vi "Report.vi"() -> ()   [LabVIEW 2017]
uses:
  <vilib>/Utility/miscctls.llb/LVRowAndColumnUnsignedTypeDef.ctl
  a160b8e7-0040-4e34-a052-5f80b3aab475.vi
  <vilib>/addons/database/Connection.llb/DB Tools Open Connec (String).vi
  <vilib>/Utility/file.llb/Write Delimited Spreadsheet (string).vi
  Global/Global 1.vi
  <vilib>/regexp/Match Regular Expression.xnode
  <vilib>/addons/database/NI_Database_API.lvlib
  <vilib>/Utility/NIReport.llb/NI_report.lvclass
  <vilib>/Utility/NIReport.llb/Append Text Table to Report (wrap).vi
  <vilib>/Utility/miscctls.llb/LVRowAndColumnTypeDef.ctl
panel:
  out "reposr save header":string[](array[string])
  in  "SELECT REPORT TYPE":string(combo)="WITH TRECIABILITY"
  out "error out":errorcluster
  in  "error in (no error)":errorcluster
  in  "GET REPORT":bool
  in  "EXIT":bool
  in  "EXPORT TO EXCEL":bool
  in  "TO":timestamp format="%<%x>T"
  in  "FROM":timestamp format="%<%x>T"
  in  "BARCODE":string
  in  "TYPE":string(combo)="DATE TIME"
  in  "STATION WISE":string(combo)="0"
  out "Table":string[][](table)
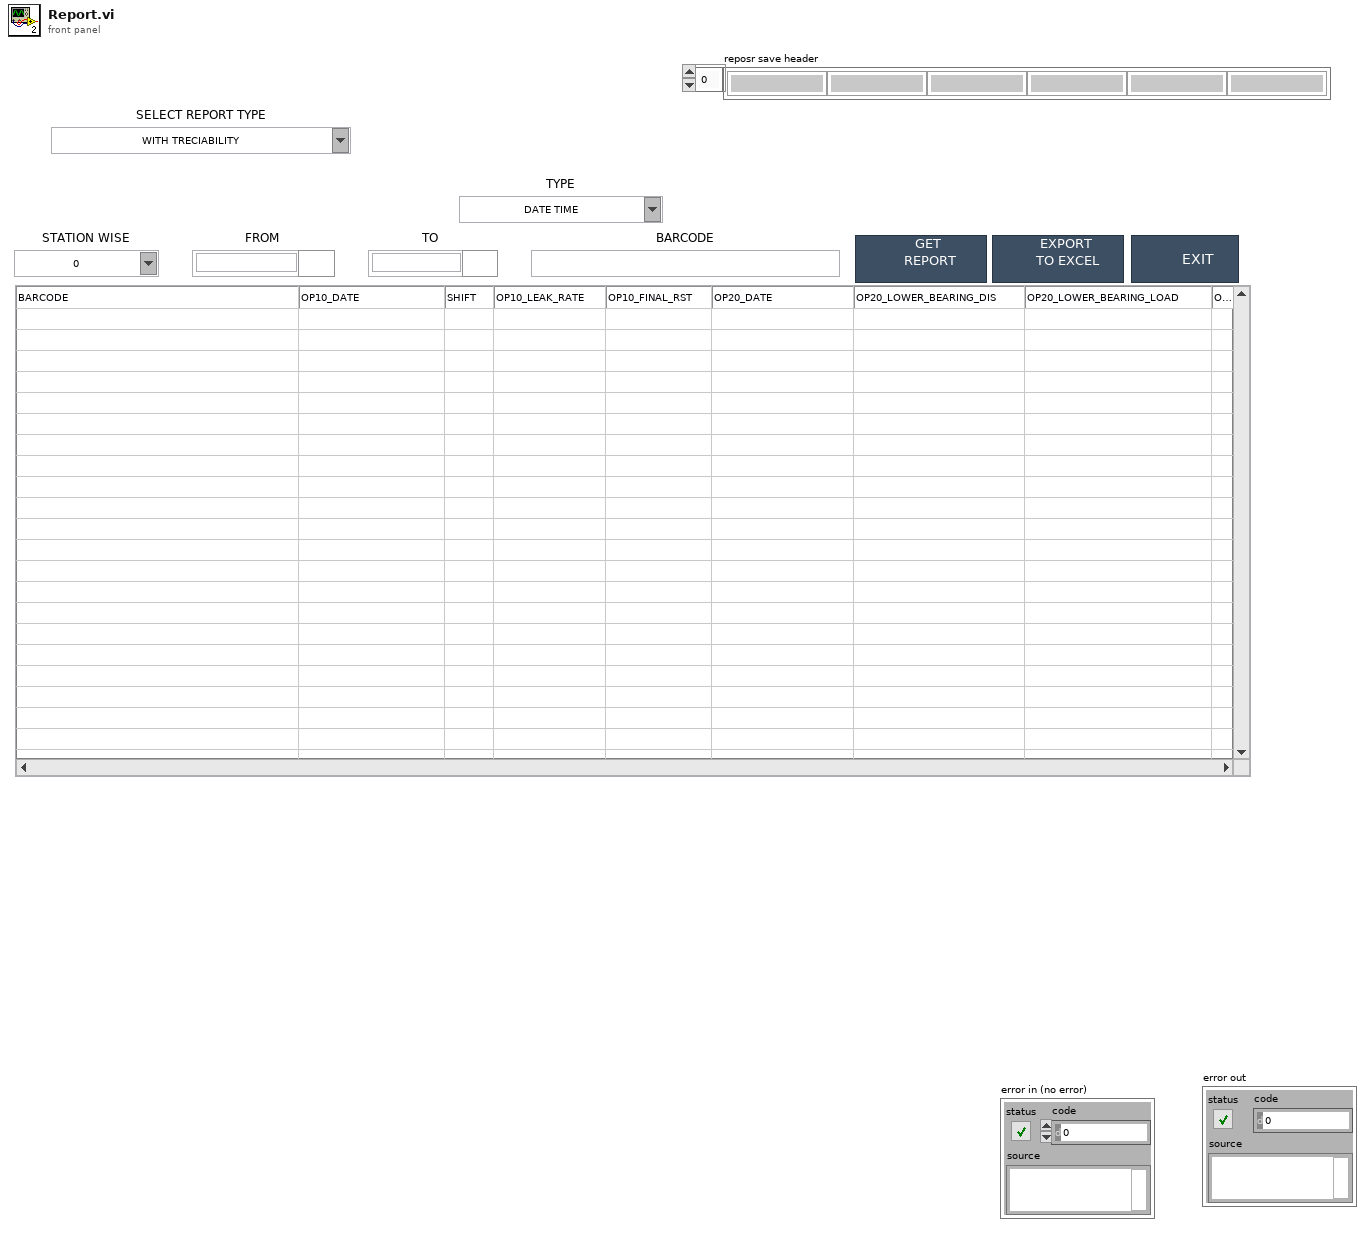
[diagram p1: front panel]
types:
  T1 = typedef "NI_Database_API.lvlib/Conn ObjectReference.ctl" = refnum<k1>
  T2 = typedef "LVRowAndColumnTypeDef.ctl" = cluster{"Row":i32, "Column":i32}
  T3 = typedef "LVRowAndColumnUnsignedTypeDef.ctl" = cluster{"Row":u32, "Column":u32}
  T4 = enum16{"Standard Report", "HTML", "Word", "Excel"}
  T5 = enum16{"maximized", "minimized", "normal", "no change"}
  T6 = enum32{"invalid app kind", "Development System", "Run Time System", "Student Edition", "Embedded LabVIEW", "Evaluation", "Custom"}
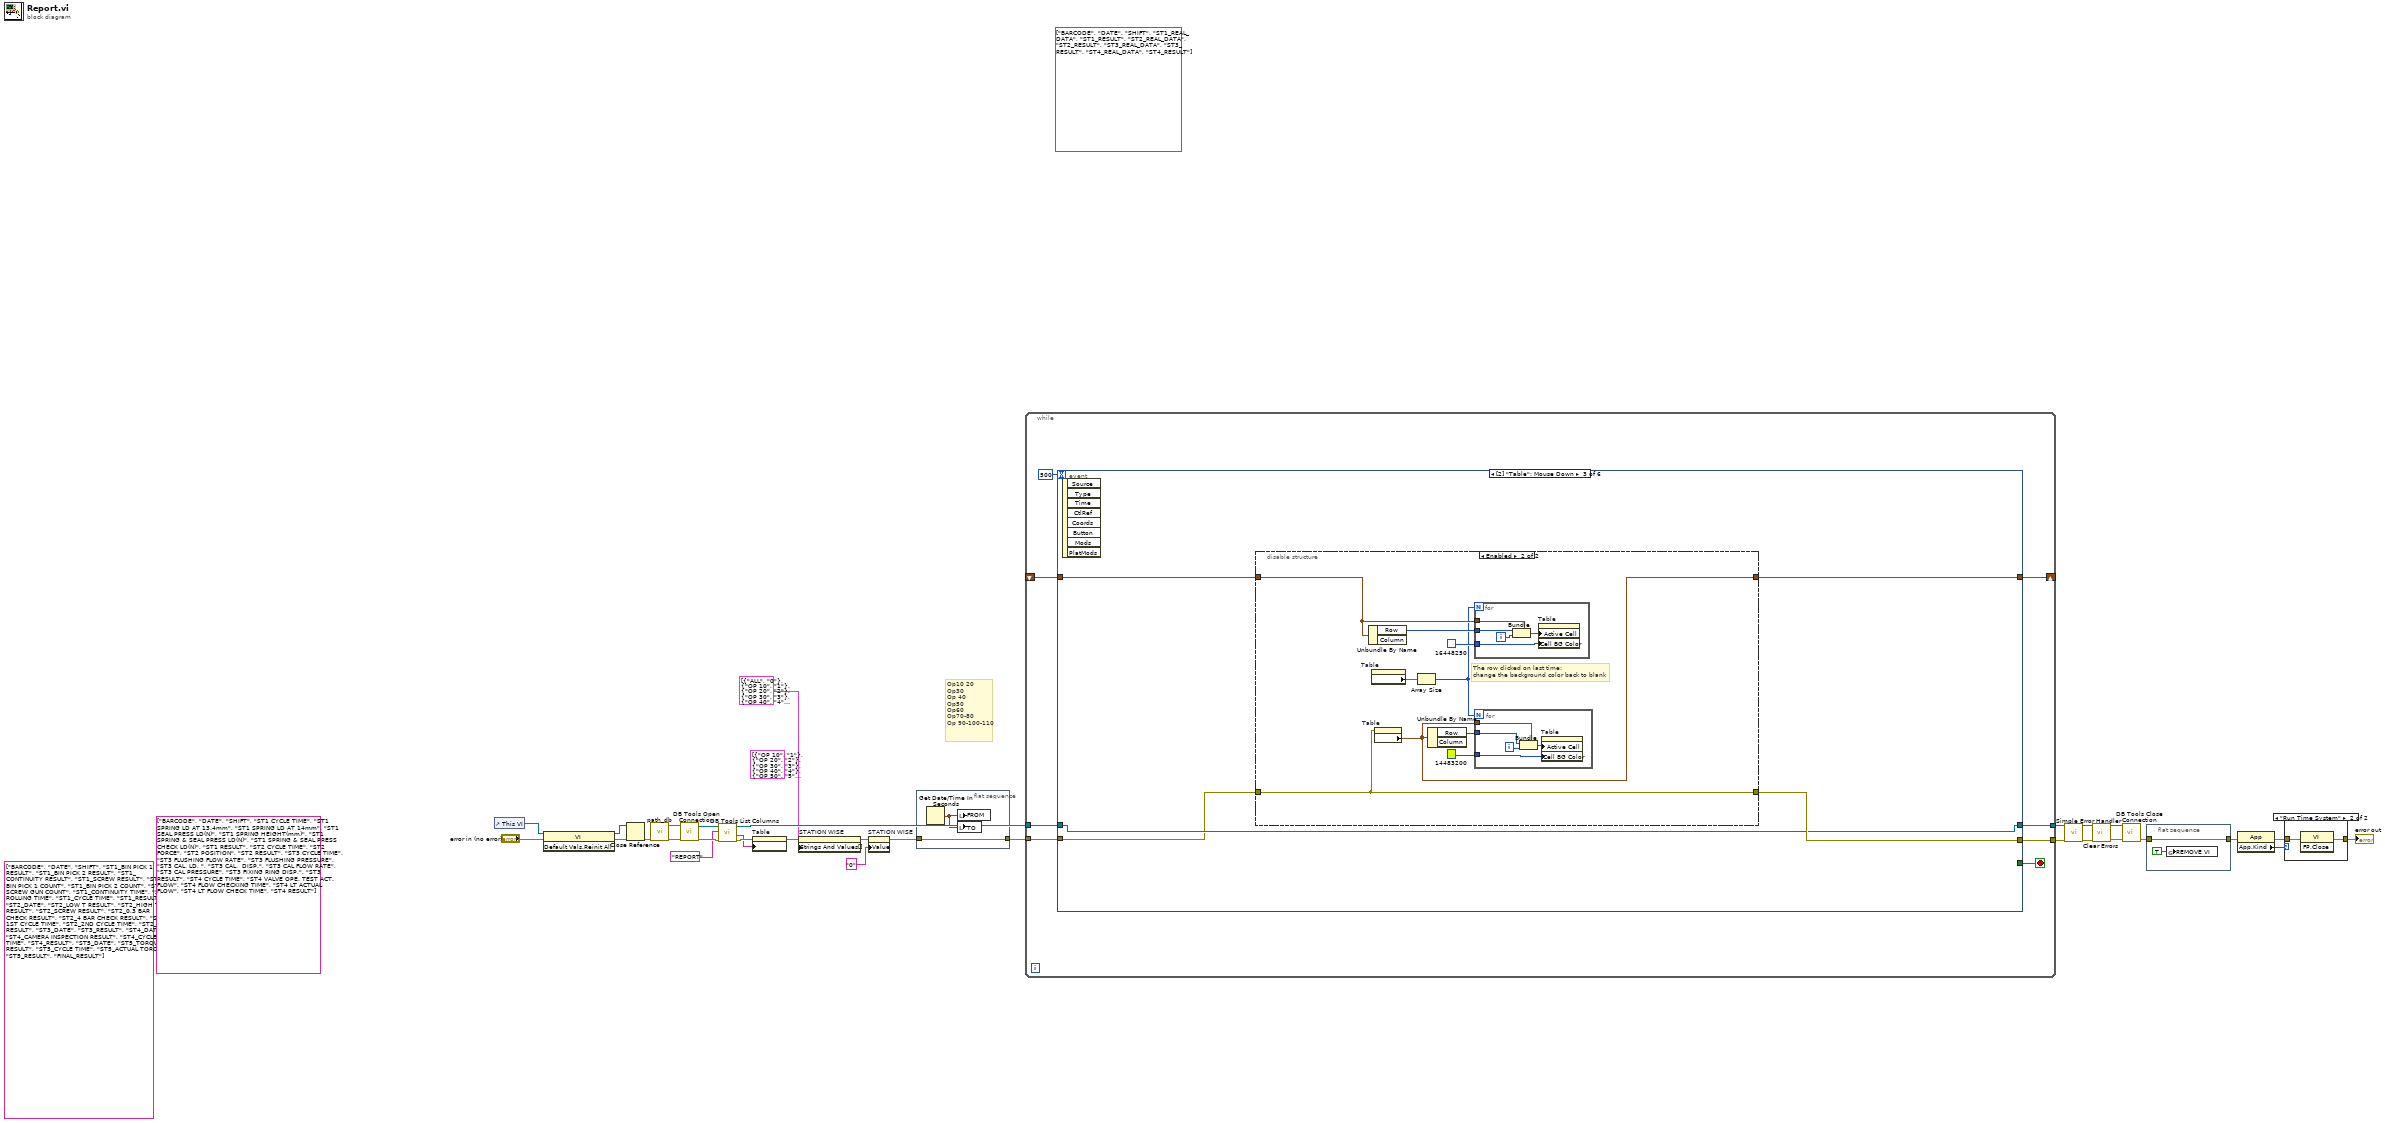
[diagram p0: block diagram]
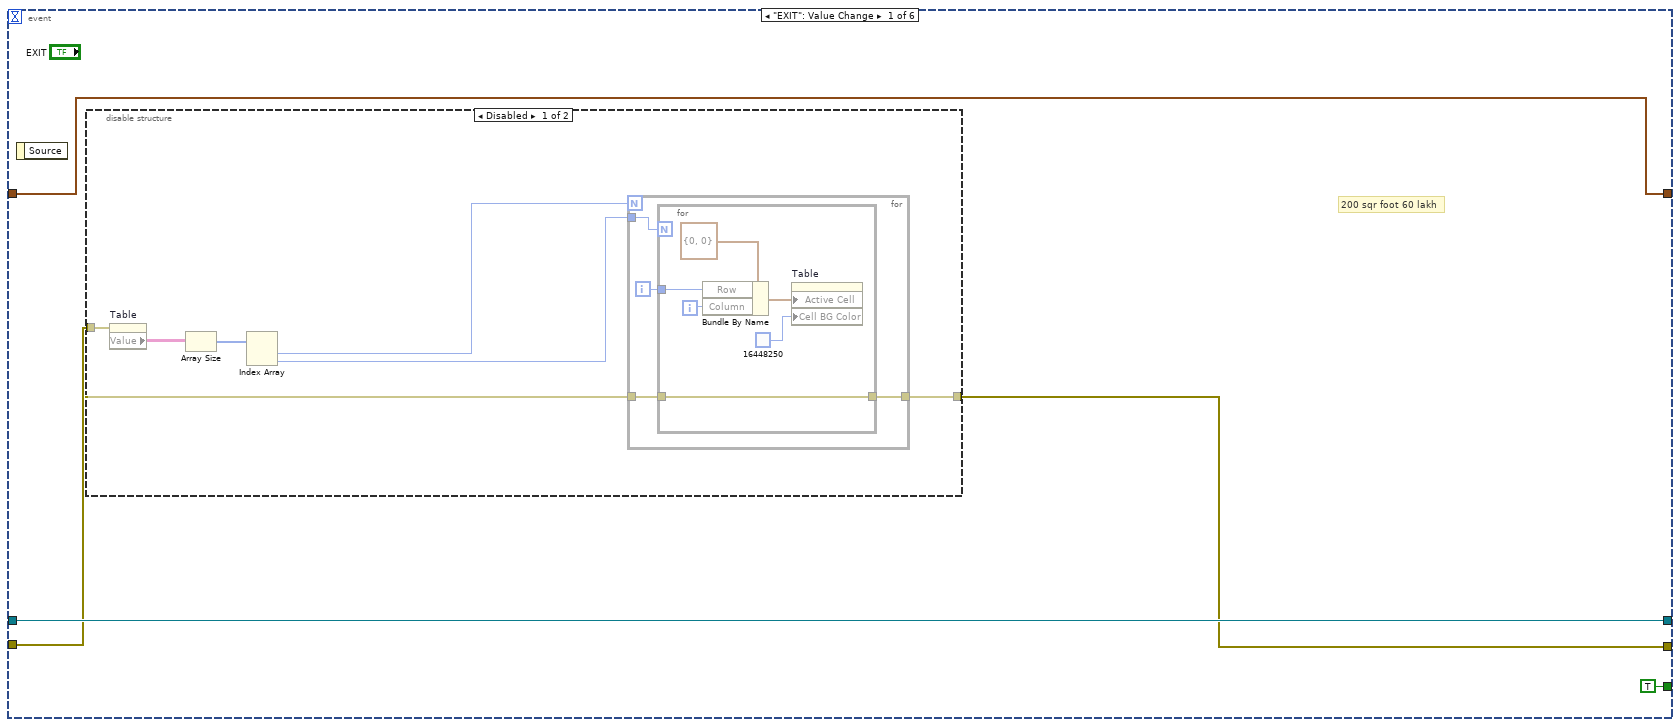
[diagram p2: hidden frame]
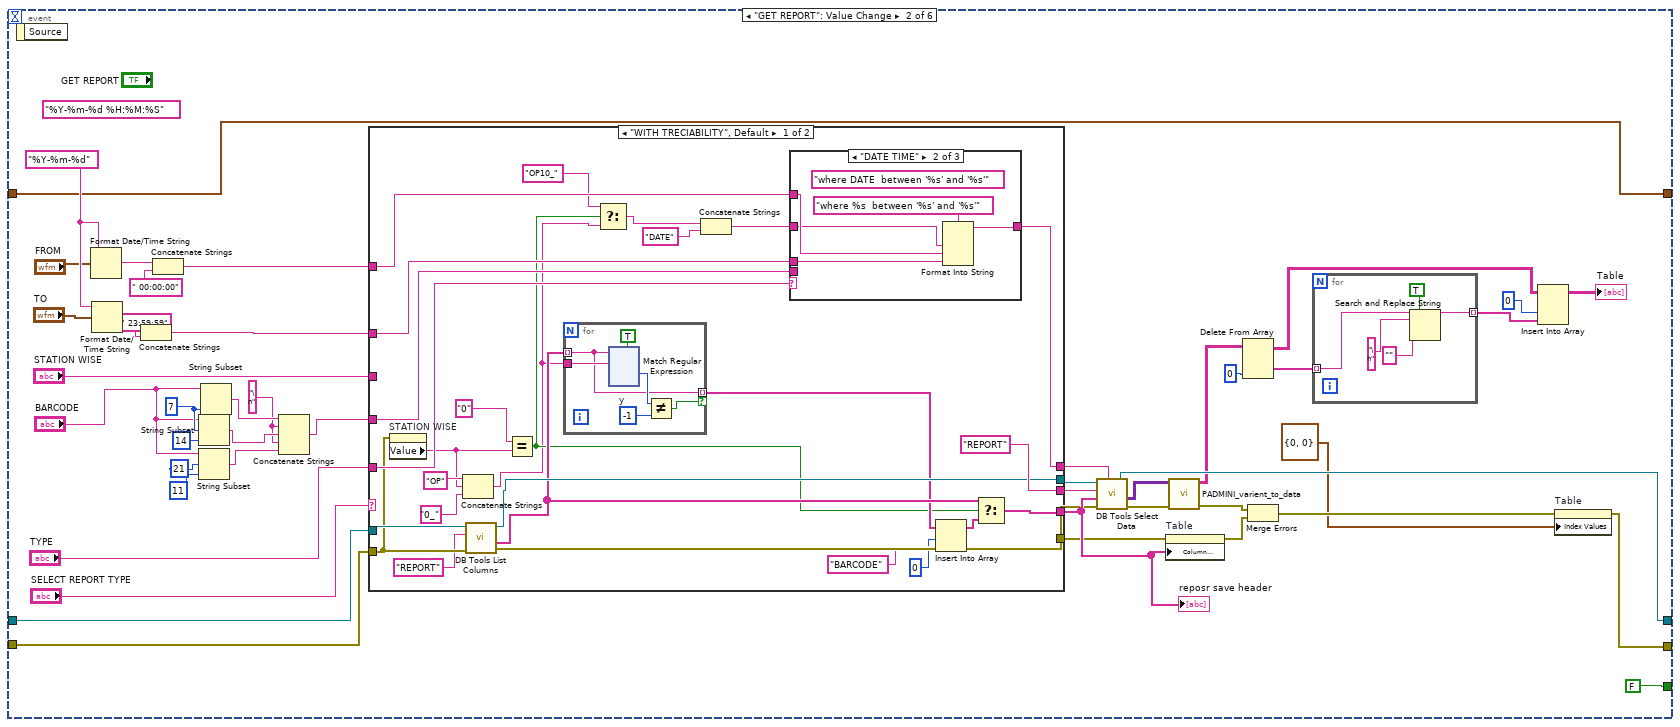
[diagram p4: hidden frame]
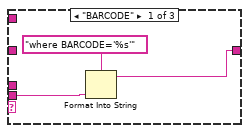
[diagram p5: hidden frame]
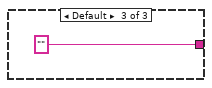
[diagram p6: hidden frame]
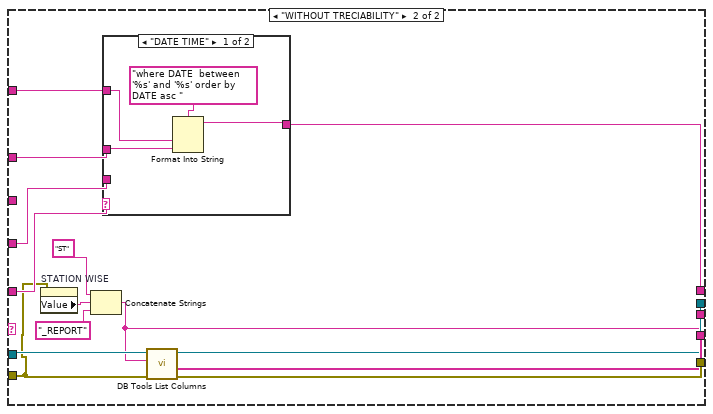
[diagram p7: hidden frame]
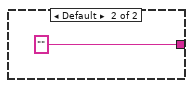
[diagram p8: hidden frame]
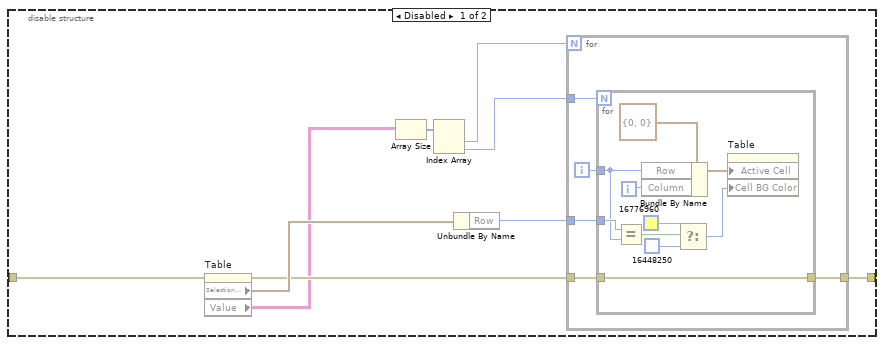
[diagram p9: hidden frame]
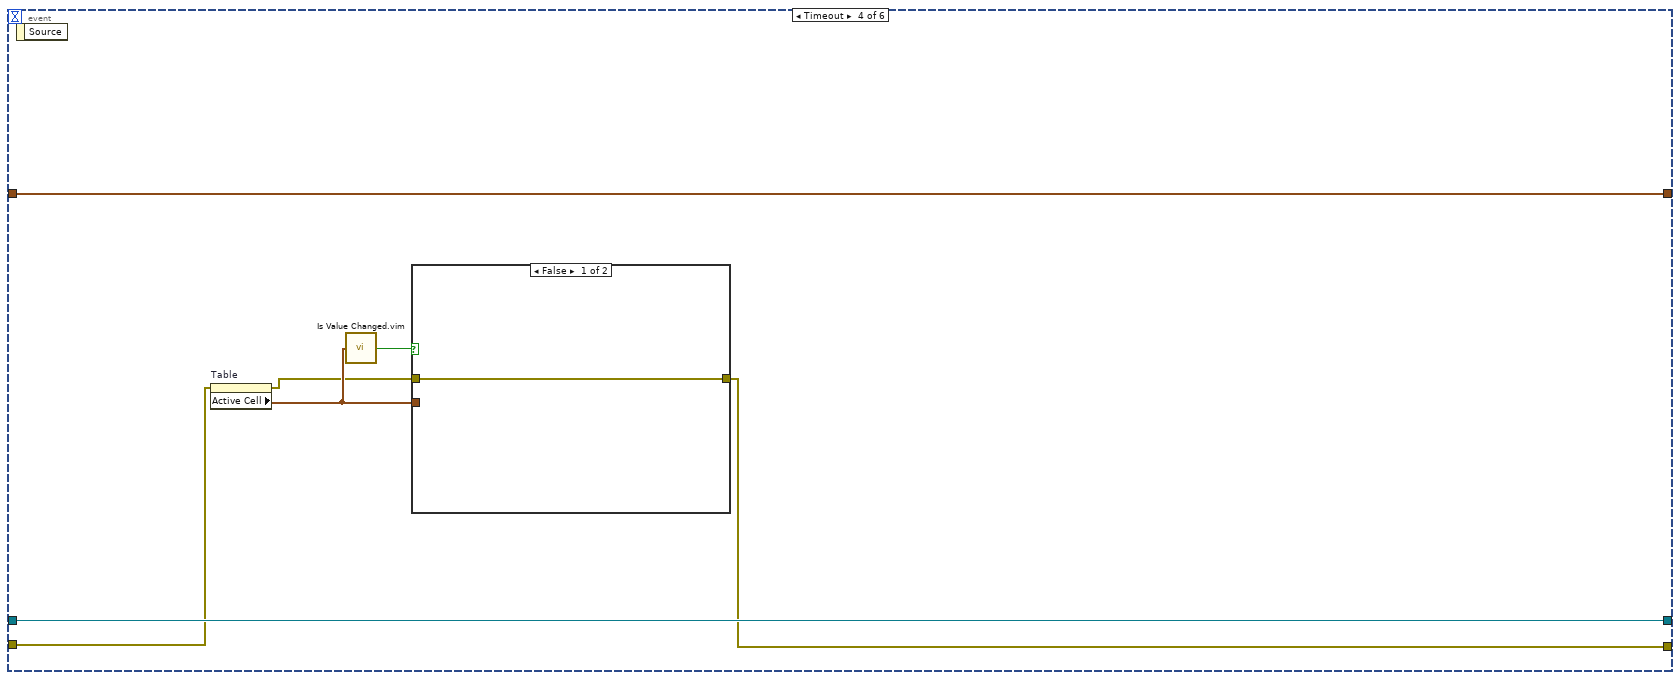
[diagram p10: hidden frame]
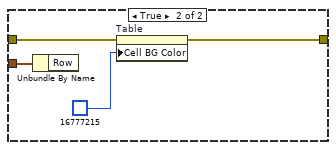
[diagram p11: hidden frame]
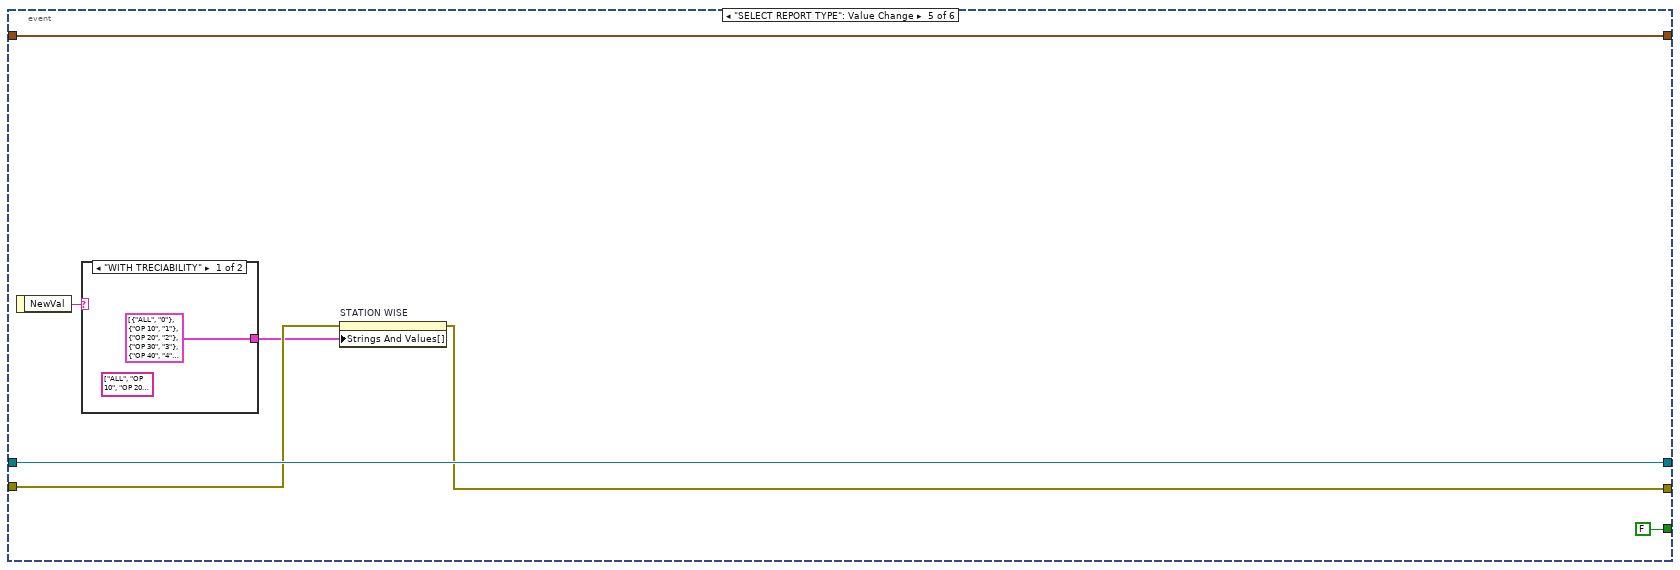
[diagram p12: hidden frame]
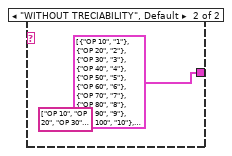
[diagram p13: hidden frame]
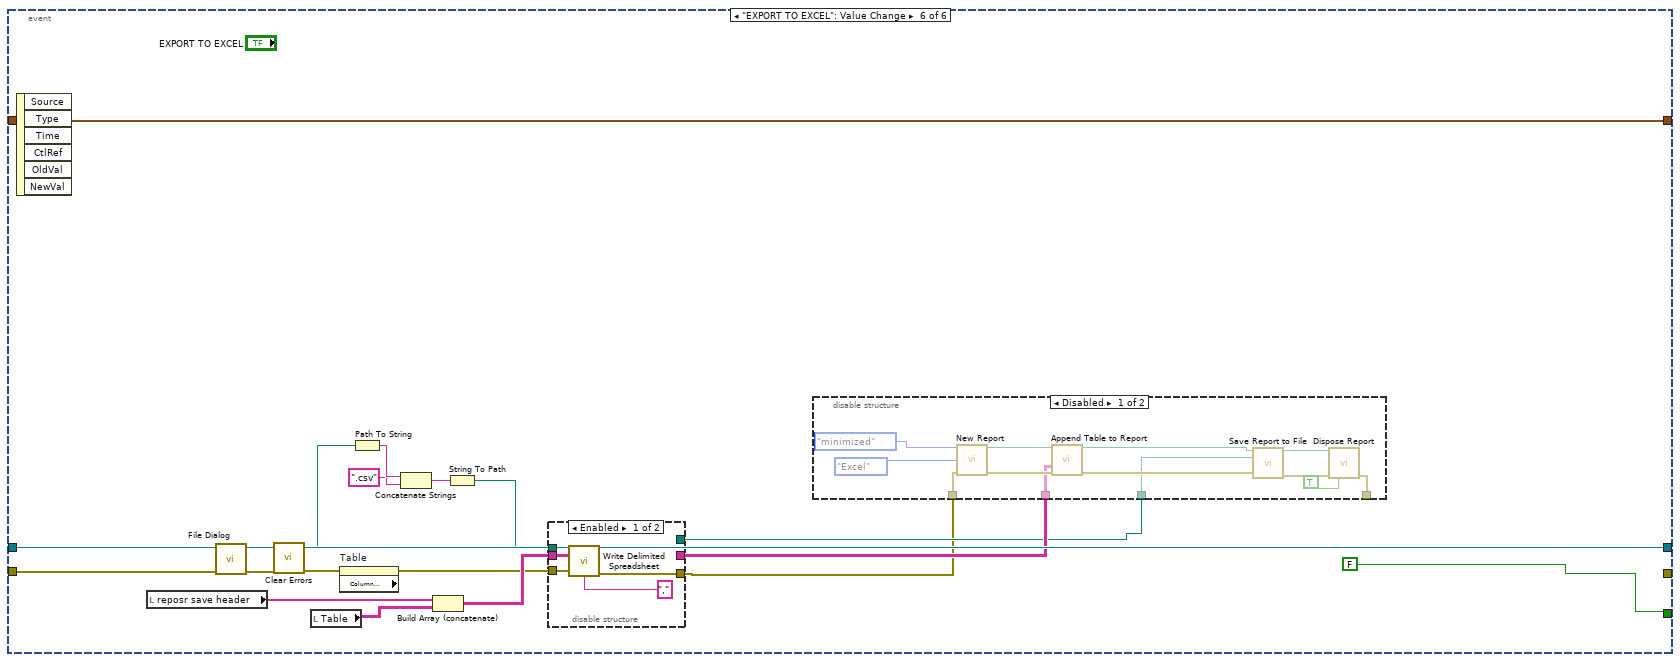
[diagram p14: hidden frame]
diagram:
  (unwired) cluster{"String":string, "Value":string}[] [{"String"="OP 10", "Value"="1"}, {"String"="OP 20", "Value"="2"}, {"String"="OP 30", "Value"="3"}, {"String"="OP 40", "Value"="4"}, {"String"="OP 50", "Value"="5"}, {"String"="OP 60", "Value"="6"}, {"String"="OP 70", "Value"="7"}, {"String"="OP 80", "Value"="8"}, {"String"="OP 90", "Value"="9"}, {"String"="OP 100", "Value"="10"}, {"String"="OP 110", "Value"="11"}] ("Strings And Values [] 2")
  (unwired) string[] ["BARCODE", "DATE", "SHIFT", "ST1_REAL_DATA", "ST1_RESULT", "ST2_REAL_DATA", "ST2_RESULT", "ST3_REAL_DATA", "ST3_RESULT", "ST4_REAL_DATA", "ST4_RESULT"]
  (unwired) string[] ["BARCODE", "DATE", "SHIFT", "ST1_BIN PICK 1 RESULT", "ST1_BIN PICK 2 RESULT", "ST1_CONTINUITY RESULT", "ST1_SCREW RESULT", "ST1_BIN PICK 1 COUNT", "ST1_BIN PICK 2 COUNT", "ST1_SCREW GUN COUNT", "ST1_CONTINUITY TIME", "ST1_ROLLING TIME", "ST1_CYCLE TIME", "ST1_RESULT", "ST2_DATE", "ST2_LOW T RESULT", "ST2_HIGH T RESULT", "ST2_SCREW RESULT", "ST2_0.3 BAR CHECK RESULT", "ST2_4 BAR CHECK RESULT", "ST2_1ST CYCLE TIME", "ST2_2ND CYCLE TIME", "ST2_RESULT", "ST3_DATE", "ST3_RESULT", "ST4_DATE", "ST4_CAMERA INSPECTION RESULT", "ST4_CYCLE TIME", "ST4_RESULT", "ST5_DATE", "ST5_TORQUE RESULT", "ST5_CYCLE TIME", "ST5_ACTUAL TORQUE", "ST5_RESULT", "FINAL_RESULT"]
  (unwired) string[] ["BARCODE", "DATE", "SHIFT", "ST1 CYCLE TIME", "ST1 SPRING LD AT 13.4mm", "ST1 SPRING LD AT 14mm", "ST1 SEAL PRESS LD(N)", "ST1 SPRING HEIGHT(mm)", "ST1 SPRING & SEAL PRESS LD(N)", "ST1 SPRING & SEAL PRESS CHECK LD(N)", "ST1 RESULT", "ST2 CYCLE TIME", "ST2 FORCE", "ST2 POSITION", "ST2 RESULT", "ST3 CYCLE TIME", "ST3 FLUSHING FLOW RATE", "ST3 FLUSHING PRESSURE", "ST3 CAL. LD. ", "ST3 CAL.  DISP.", "ST3 CAL FLOW RATE", "ST3 CAL PRESSURE", "ST3 FIXING RING DISP.", "ST3 RESULT", "ST4 CYCLE TIME", "ST4 VALVE OPE. TEST ACT. FLOW", "ST4 FLOW CHECKING TIME", "ST4 LT ACTUAL FLOW", "ST4 LT FLOW CHECK TIME", "ST4 RESULT"]
  # "Op10 20\nOp30\nOp 40\nOp50\nOp60\nOp70-80\nOp 90-100-110"
  n1 = control-ref of="This VI"() -> (w28:refnum<vi>)
  n2 = invoke class="VI" method="Default Vals.Reinit All"(reference=w28, error in="error in (no error)") -> (reference out=w26:refnum<vi>, error out=w25:errorcluster)  [unwired: 1 in, 1 out]
  n3 = Close Reference(reference=w26, error in (no error)=w25) -> (error out=w16:errorcluster)
  n4 = call "path_db.vi"("error in"=w16) -> ("error out"=w18:errorcluster, "resulting string"=w17:string)  [unwired: 9 in]
  n5 = call-poly <vilib>:"DB Tools Open Connection.vi"("error in (no error)"=w18, "connection information"=w17) -> ("error out"=w11:errorcluster, "connection reference"=w8:T1)  [unwired: 6 in]
  n6 = call <vilib>:"DB Tools List Columns.vi"("error in (no error)"=w11, "table"="REPORT", "connection reference"=w8) -> ("error out"=w10:errorcluster, "columns"=w7:string[], "connection reference out"=w9:T1)  [unwired: 1 in, 1 out]
  n7 = property on="Table" class="Tbl (strict)"(error in=w10, "Column Headers[]"=w7) -> (error out=w13:errorcluster)  [unwired: 1 in, 1 out]
  n8 = property on="STATION WISE" class="CmbBox"(error in=w13, "Strings And Values[]"=cluster{"String":string, "Value":string}[] [{"String"="ALL", "Value"="0"}, {"String"="OP 10", "Value"="1"}, {"String"="OP 20", "Value"="2"}, {"String"="OP 30", "Value"="3"}, {"String"="OP 40", "Value"="4"}, {"String"="OP 50", "Value"="5"}, {"String"="OP 60", "Value"="6"}, {"String"="OP 70", "Value"="7"}, {"String"="OP 80", "Value"="8"}, {"String"="OP 90", "Value"="9"}, {"String"="OP 100", "Value"="10"}, {"String"="OP 110", "Value"="11"}] ("Strings And Values [] 2")) -> (error out=w5:errorcluster)  [unwired: 1 in, 1 out]
  n9 = property on="STATION WISE" class="CmbBox"(error in=w5, "Value"="0") -> (error out=w4:errorcluster)  [unwired: 1 in, 1 out]
  n10 = flat-sequence {
    tunnel: w4 -> [w29]
    tunnel: [w29] -> w12
    frame #0 {
      n11 = Get Date/Time In Seconds() -> (seconds since 1Jan1904=w30:timestamp)
      n12 = local write "FROM"(w30) -> ()
      n13 = local write "TO"(w30) -> ()
    }
  }
  n14 = while {
    tunnel: [w35] -> w1
    tunnel: w12 -> [w37]
    tunnel: w9 -> [w36]
    tunnel: [w34] -> w14
    shift-right: [w32] -> _
    shift-left: _ -> [w31]
    stop <- w38 stop-if-true
    n15 = event shown="[2] \"Table\": Mouse Down" {
      selector: _ -> [_ _ _ _ _ _]
      dyn-events: _ -> [_ _ _ _ _ _]
      timeout: 500 -> [_ _ _ _ _ _]
      tunnel: [TRUE FALSE _ _ FALSE FALSE] -> w38
      tunnel: w37 -> [w41 w84 w288 w337 w350 w360]
      tunnel: w36 -> [w42 w82 w289 w340 w352 w371]
      tunnel: [w42 w90 w289 w340 w352 w371] -> w34
      tunnel: [w40 w71 w290 w335 w347 _] -> w35
      tunnel: [w39 w70 w287 w334 w346 w355] -> w32
      tunnel: w31 -> [w39 w70 w286 w334 w346 w355]
      event "EXIT": Value Change {
        # "200 sqr foot 60 lakh"
        n16 = event-data() -> ()  [unwired: 1 in, 1 out]
        n17 = disable-structure shown="Disabled" {
          disable-tunnel: w41 -> [w49 _]
          disable-tunnel: [w48 _] -> w40
          frame Disabled {
            n18 = property on="Table" class="Tbl (strict)"(error in=w49) -> ("Value"=w47:string[][])  [unwired: 1 in, 2 out]
            n19 = Array Size(array=w47) -> (size(s)=w46:i32[])
            n20 = Index Array(array=w46) -> (element #1=w45:i32, element #2=w44:i32)  [unwired: 2 in]
            n21 = for {
              N: w45 -> [_]
              tunnel: w44 -> [w53]
              tunnel: [w50] -> w48
              tunnel: w49 -> [w51]
              i -> [w52]
              n22 = for {
                N: w53 -> [_]
                tunnel: w52 -> [w56]
                tunnel: w51 -> [w55]
                tunnel: [w55] -> w50
                i -> [w57]
                n23 = Bundle By Name(cluster=T2 {"Row"=0, "Column"=0} ("Selection Start 2"), "Row"=w56, "Column"=w57) -> (w58:T2)
                n24 = property on="Table" class="Tbl (strict)"("Active Cell"=w58, "Cell BG Color"=u32 16448250) -> ()  [unwired: 2 in, 2 out]
              }
            }
          }
          frame Enabled {
          }
        }
      }
      event "GET REPORT": Value Change {
        w62 = "\n"
        w69 = 7 ("line index")
        (unwired) "%Y-%m-%d %H:%M:%S" ("time format string (%c)")
        w103 = "%Y-%m-%d" ("time format string (%c)")
        n25 = event-data() -> ()  [unwired: 1 in, 1 out]
        n26 = Format Date/Time String(time format string (%c)=w103, seconds (now)="FROM") -> (date/time string=w97:string)  [unwired: 1 in]
        n27 = Format Date/Time String(time format string (%c)=w103, seconds (now)="TO") -> (date/time string=w94:string)  [unwired: 1 in]
        n28 = Concatenate Strings(w94, " 23:59:59" ("time format string (%c)")) -> (w93:string)
        n29 = Concatenate Strings(w97, " 00:00:00" ("time format string (%c)")) -> (w96:string)
        n30 = String Subset(string="BARCODE", offset (0)=w69, length (rest)=14 ("line index")) -> (substring=w64:string)
        n31 = String Subset(string="BARCODE", offset (0)=21 ("line index"), length (rest)=11 ("line index")) -> (substring=w63:string)
        n32 = String Subset(string="BARCODE", length (rest)=w69) -> (substring=w65:string)  [unwired: 1 in]
        n33 = Concatenate Strings(w65, w62, w64, w62, w63) -> (w61:string)
        n34 = case shown="\"WITH TRECIABILITY\", Default" "SELECT REPORT TYPE" {
          tunnel: "TYPE" -> [w137 w280]
          tunnel: [w136 w279] -> w104
          tunnel: w61 -> [w135 w278]
          tunnel: w96 -> [w134 w277]
          tunnel: w93 -> [w119 w273]
          tunnel: "STATION WISE" -> [_ _]
          tunnel: ["REPORT" w268] -> w85
          tunnel: w84 -> [w125 w267]
          tunnel: [w130 w272] -> w79
          tunnel: [w117 w271] -> w83
          tunnel: w82 -> [w132 w270]
          tunnel: [w131 w269] -> w81
          frame "WITH TRECIABILITY", Default {
            n35 = property on="STATION WISE" class="CmbBox"(error in=w125) -> ("Value"=w120:string)  [unwired: 1 in, 2 out]
            n36 = Concatenate Strings("OP" ("element"), w120, "0_" ("element")) -> (w112:string)
            n37 = call <vilib>:"DB Tools List Columns.vi"("error in (no error)"=w125, "table"="REPORT", "connection reference"=w132) -> ("error out"=w130:errorcluster, "columns"=w124:string[], "connection reference out"=w131:T1)  [unwired: 1 in, 1 out]
            n38 = Equal?(x="0", y=w120) -> (x = y?=w114:bool)
            n39 = for {
              tunnel: w124 -> [w139] mode=indexing
              tunnel: w112 -> [w143]
              tunnel: [w139] -> w118 mode=indexing if=w138
              w140 = -1  # y
              n40 = xnode "Match Regular Expression"("input string"=w139, "regular expression"=w143, "multiline? (F)"=TRUE) -> ("offset past match"=w141:i32)  [unwired: 3 in, 4 out]
              n41 = Not Equal?(x=w141, y=w140) -> (x != y?=w138:bool)
            }
            n42 = Select(t="OP10_", s=w114, f=w112) -> (s? t:f=w111:string)
            n43 = Concatenate Strings(w111, "DATE") -> (w115:string)
            n44 = case shown="\"DATE TIME\"" w137 {
              tunnel: [w259 w264 ""] -> w136
              tunnel: w135 -> [w258 _ _]
              tunnel: w134 -> [_ w263 _]
              tunnel: w119 -> [_ w262 _]
              tunnel: w115 -> [_ w261 _]
              frame "BARCODE" {
                n45 = Format Into String(format string="where BARCODE='%s'", w258) -> (resulting string=w259:string)  [unwired: 2 in, 1 out]
              }
              frame "DATE TIME" {
                (unwired) "where DATE  between '%s' and '%s'"
                n46 = Format Into String(format string="where %s  between '%s' and '%s'", w261, w263, w262) -> (resulting string=w264:string)  [unwired: 2 in, 1 out]
              }
              frame Default {
              }
            }
            n47 = Insert Into Array(array=w118, index=0, new element="BARCODE" ("String")) -> (w128:string[])
            n48 = Select(t=w124, s=w114, f=w128) -> (s? t:f=w117:string[])
          }
          frame "WITHOUT TRECIABILITY" {
            n49 = property on="STATION WISE" class="CmbBox"(error in=w267) -> ("Value"=w276:string)  [unwired: 1 in, 2 out]
            n50 = Concatenate Strings("ST", w276, "_REPORT") -> (w268:string)
            n51 = case shown="\"DATE TIME\"" w280 {
              tunnel: [w284 ""] -> w279
              tunnel: w278 -> [_ _]
              tunnel: w277 -> [w283 _]
              tunnel: w273 -> [w282 _]
              frame "DATE TIME" {
                n52 = Format Into String(format string="where DATE  between '%s' and '%s' order by DATE asc ", w283, w282) -> (resulting string=w284:string)  [unwired: 2 in, 1 out]
              }
              frame Default {
              }
            }
            n53 = call <vilib>:"DB Tools List Columns.vi"("error in (no error)"=w267, "table"=w268, "connection reference"=w270) -> ("error out"=w272:errorcluster, "columns"=w271:string[], "connection reference out"=w269:T1)  [unwired: 1 in, 1 out]
          }
        }
        "reposr save header" <- w83
        n54 = call <vilib>:"DB Tools Select Data.vi"("condition"=w104, "error in (no error)"=w79, "columns"=w83, "table"=w85, "connection reference"=w81) -> ("error out"=w88:errorcluster, "data"=w92:variant[][], "connection reference out"=w90:T1)  [unwired: 1 in]
        n55 = property on="Table" class="Tbl (strict)"(error in=w79, "Column Headers[]"=w83) -> (error out=w87:errorcluster)  [unwired: 1 in, 1 out]
        n56 = call "PADMINI_varient_to_data.vi"("error in (no error)"=w88, "data"=w92) -> ("error out"=w86:errorcluster, "Array"=w74:string[][])  [unwired: 8 in]
        n57 = Delete From Array(array=w74, index (col)=0 ("disabled index (col)")) -> (deleted portion=w77:string[], array with subset deleted=w75:string[][])  [unwired: 2 in]
        n58 = Merge Errors(w86, w87) -> (w91:errorcluster)
        n59 = for {
          tunnel: w77 -> [w107] mode=indexing
          tunnel: [w106] -> w76 mode=indexing
          n60 = Search and Replace String(replace all?=TRUE ("replace all? (F)"), input string=w107, search string="\n", replace string="" ("replace string (\"\")")) -> (result string=w106:string)  [unwired: 4 in, 3 out]
        }
        n61 = Insert Into Array(array=w75, index (col)=0 ("disabled index (col)"), new element=w76) -> (→"Table":string[][])  [unwired: 1 in]
        n62 = property on="Table" class="Tbl (strict)"(error in=w91, "Index Values"=T3 {"Row"=0, "Column"=0}) -> (error out=w71:errorcluster)  [unwired: 1 in, 1 out]
      }
      event "Table": Mouse Down {
        n63 = event-data() -> ()  [unwired: 1 in, 8 out]
        n64 = disable-structure shown="Enabled" {
          disable-tunnel: [w299 w317] -> w290
          disable-tunnel: w288 -> [w296 w317]
          disable-tunnel: [_ w318] -> w287
          disable-tunnel: w286 -> [_ w319]
          frame Disabled {
            n65 = property on="Table" class="Tbl (strict)"(error in=w296) -> (error out=w295:errorcluster, "Selection Start"=w297:T2, "Value"=w293:string[][])  [unwired: 1 in, 1 out]
            n66 = Array Size(array=w293) -> (size(s)=w294:i32[])
            n67 = Index Array(array=w294) -> (element #1=w291:i32, element #2=w292:i32)  [unwired: 2 in]
            n68 = Unbundle By Name(w297) -> ("Row"=w298:i32)
            n69 = for {
              N: w291 -> [_]
              tunnel: w298 -> [w302]
              tunnel: w292 -> [w304]
              tunnel: [w300] -> w299
              tunnel: w295 -> [w301]
              i -> [w303]
              n70 = for {
                N: w304 -> [_]
                tunnel: w303 -> [w310]
                tunnel: w302 -> [w311]
                tunnel: w301 -> [w305]
                tunnel: [w305] -> w300
                i -> [w312]
                n71 = Equal?(x=w311, y=w310) -> (x = y?=w309:bool)
                n72 = Bundle By Name(cluster=T2 {"Row"=0, "Column"=0} ("Selection Start 2"), "Row"=w310, "Column"=w312) -> (w313:T2)
                n73 = Select(t=u32 16776960, s=w309, f=u32 16448250) -> (s? t:f=w306:u32)
                n74 = property on="Table" class="Tbl (strict)"("Active Cell"=w313, "Cell BG Color"=w306) -> ()  [unwired: 2 in, 2 out]
              }
            }
          }
          frame Enabled {
            # "The row clicked on last time:\nchange the background color back to blank"
            n75 = Unbundle By Name(w319) -> ("Row"=w321:i32)  [unwired: 1 out]
            n76 = property on="Table" class="Tbl (strict)"() -> ("Column Headers[]"=w316:string[])  [unwired: 2 in, 2 out]
            n77 = property on="Table" class="Tbl (strict)"(error in=w317) -> ("Selection Start"=w318:T2)  [unwired: 1 in, 2 out]
            n78 = Array Size(array=w316) -> (size(s)=w315:i32)
            n79 = Unbundle By Name(w318) -> ("Row"=w322:i32)  [unwired: 1 out]
            n80 = for {
              N: w315 -> [_]
              tunnel: u32 16448250 -> [w328]
              tunnel: w319 -> [w327]
              tunnel: w321 -> [w326]
              i -> [w325]
              n81 = Bundle(cluster=w327, "Row"=w326, "Column"=w325) -> (w324:T2)
              n82 = property on="Table" class="Tbl (strict)"("Active Cell"=w324, "Cell BG Color"=w328) -> ()  [unwired: 2 in, 2 out]
            }
            n83 = for {
              N: w315 -> [_]
              tunnel: u32 14483200 -> [w333]
              tunnel: w318 -> [w332]
              tunnel: w322 -> [w331]
              i -> [w330]
              n84 = Bundle(cluster=w332, "Row"=w331, "Column"=w330) -> (w329:T2)
              n85 = property on="Table" class="Tbl (strict)"("Active Cell"=w329, "Cell BG Color"=w333) -> ()  [unwired: 2 in, 2 out]
            }
          }
        }
      }
      event Timeout {
        n86 = event-data() -> ()  [unwired: 1 in, 1 out]
        n87 = property on="Table" class="Tbl (strict)"(error in=w337) -> (error out=w336:errorcluster, "Active Cell"=w339:T2)  [unwired: 1 in, 1 out]
        n88 = call "Is Value Changed.vim"("value"=w339) -> ("changed or first call?"=w338:bool)
        n89 = case shown="False" w338 {
          tunnel: w339 -> [_ w345]
          tunnel: w336 -> [w341 w343]
          tunnel: [w341 w342] -> w335
          frame False {
          }
          frame True {
            n90 = Unbundle By Name(w345) -> ()  [unwired: 1 out]
            n91 = property on="Table" class="Tbl (strict)"(error in=w343, "Cell BG Color"=u32 16777215) -> (error out=w342:errorcluster)  [unwired: 1 in, 1 out]
          }
        }
      }
      event "SELECT REPORT TYPE": Value Change {
        n92 = event-data() -> ("NewVal"=w351:string)  [unwired: 1 in]
        n93 = case shown="\"WITH TRECIABILITY\"" w351 {
          tunnel: [cluster{"String":string, "Value":string}[] [{"String"="ALL", "Value"="0"}, {"String"="OP 10", "Value"="1"}, {"String"="OP 20", "Value"="2"}, {"String"="OP 30", "Value"="3"}, {"String"="OP 40", "Value"="4"}, {"String"="OP 50", "Value"="5"}, {"String"="OP 60", "Value"="6"}, {"String"="OP 70", "Value"="7"}, {"String"="OP 80", "Value"="8"}, {"String"="OP 90", "Value"="9"}, {"String"="OP 100", "Value"="10"}, {"String"="OP 110", "Value"="11"}] ("Strings And Values [] 2") cluster{"String":string, "Value":string}[] [{"String"="OP 10", "Value"="1"}, {"String"="OP 20", "Value"="2"}, {"String"="OP 30", "Value"="3"}, {"String"="OP 40", "Value"="4"}, {"String"="OP 50", "Value"="5"}, {"String"="OP 60", "Value"="6"}, {"String"="OP 70", "Value"="7"}, {"String"="OP 80", "Value"="8"}, {"String"="OP 90", "Value"="9"}, {"String"="OP 100", "Value"="10"}, {"String"="OP 110", "Value"="11"}] ("Strings And Values [] 2")] -> w348
          frame "WITH TRECIABILITY" {
            (unwired) string[] ["ALL", "OP 10", "OP 20", "OP 30", "OP 40", "OP 50", "OP 60", "OP 70", "OP 80", "OP 90", "OP 100", "OP 110"] ("Strings []")
          }
          frame "WITHOUT TRECIABILITY", Default {
            (unwired) string[] ["OP 10", "OP 20", "OP 30", "OP 40", "OP 50", "OP 60", "OP 70", "OP 80", "OP 90", "OP 100", "OP 110"] ("Strings []")
          }
        }
        n94 = property on="STATION WISE" class="CmbBox"(error in=w350, "Strings And Values[]"=w348) -> (error out=w347:errorcluster)  [unwired: 1 in, 1 out]
      }
      event "EXPORT TO EXCEL": Value Change {
        n95 = event-data() -> ()  [unwired: 1 in, 6 out]
        n96 = local read "reposr save header"() -> (w356:string[])
        n97 = call "File Dialog"("error in"=w360) -> ("selected path"=w369:path, "error out"=w370:errorcluster)  [unwired: 11 in, 2 out]
        n98 = call <vilib>:"Clear Errors.vi"("error in (no error)"=w370) -> ("error out"=w363:errorcluster)  [unwired: 5 in, 1 out]
        n99 = local read "Table"() -> (w372:string[][])
        n100 = property on="Table" class="Tbl (strict)" props=["Column Headers[]"](error in=w363) -> (error out=w362:errorcluster)  [unwired: 1 in, 2 out]
        n101 = Path To String(path=w369) -> (string=w368:string)
        n102 = Concatenate Strings(w368, ".csv" ("string")) -> (w366:string)
        n103 = Build Array (concatenate)(w356, w372) -> (w364:string[][])
        n104 = String To Path(string=w366) -> (path=w365:path)
        n105 = disable-structure shown="Enabled" {
          disable-tunnel: w365 -> [w391 w392]
          disable-tunnel: [w390 w394] -> w357
          disable-tunnel: w364 -> [w389 w393]
          disable-tunnel: w362 -> [w387 w394]
          disable-tunnel: [_ w393] -> w359
          disable-tunnel: [_ w392] -> w358
          frame Enabled {
            n106 = call-poly <vilib>:"Write Delimited Spreadsheet.vi"("file path (dialog if empty)"=w391, "2D data"=w389, "error in (no error)"=w387, "delimiter (\\t)"="," ("delimiter (\\t)")) -> ("error out"=w390:errorcluster)  [unwired: 10 in, 1 out]
          }
          frame Disabled {
          }
        }
        n107 = disable-structure shown="Disabled" {
          disable-tunnel: w359 -> [w376 _]
          disable-tunnel: w358 -> [w375 _]
          disable-tunnel: [w374 w386] -> _
          disable-tunnel: w357 -> [w373 w386]
          frame Disabled {
            n108 = call <vilib>:"New Report.vi"("window state (normal)"=T5."minimized", "report type"=T4."Excel", "error in (no error)"=w373) -> ("report out"=w383:refnum<class "NI_report.lvclass">, "error out"=w382:errorcluster)  [unwired: 11 in]
            n109 = call-poly <vilib>:"Append Table to Report.vi"("report in"=w383, "text data"=w376, "error in (no error)"=w382) -> ("report out"=w379:refnum<class "NI_report.lvclass">, "error out"=w381:errorcluster)  [unwired: 9 in, 2 out]
            n110 = call-dynamic "Save Report to File.vi"("report in"=w379, "report file path"=w375, "error in (no error)"=w381) -> ("report out"=w378:refnum<class "NI_report.lvclass">, "error out"=w380:errorcluster)  [unwired: 11 in]
            n111 = call-dynamic "Dispose Report.vi"("report in"=w378, "error in (no error)"=w380, "close report? (T)"=TRUE) -> ("error out"=w374:errorcluster)  [unwired: 12 in]
          }
          frame Enabled {
          }
        }
      }
    }
  }
  n112 = call <vilib>:"Simple Error Handler.vi"("error in (no error)"=w1) -> ("error out"=w24:errorcluster)  [unwired: 4 in, 4 out]
  n113 = call <vilib>:"Clear Errors.vi"("error in (no error)"=w24) -> ("error out"=w23:errorcluster)  [unwired: 5 in, 1 out]
  n114 = call <vilib>:"DB Tools Close Connection.vi"("error in (no error)"=w23, "connection reference"=w14) -> ("error out"=w15:errorcluster)  [unwired: 5 in]
  n115 = flat-sequence {
    tunnel: [w396] -> w22
    tunnel: w15 -> [w396]
    frame #0 {
      n116 = global write "Global 1.vi" "REMOVE VI"(TRUE ("REMOVE VI")) -> ()
    }
  }
  n117 = property class="App"(error in=w22) -> (error out=w21:errorcluster, "App.Kind"=w20:T6)  [unwired: 1 in, 1 out]
  n118 = case shown="\"Run Time System\"" w20 {
    tunnel: w21 -> [w397 w399]
    tunnel: [w397 w398] -> w19
    frame "Development System", Default {
    }
    frame "Run Time System" {
      n119 = invoke class="VI" method="FP.Close"(error in=w399) -> (error out=w398:errorcluster)  [unwired: 2 in, 2 out]
    }
  }
  "error out" <- w19
